vi "Write Configuration File.vi"(8 "error in (no error)":errorcluster, 11 "Inst.RP100 in":refnum<class "Inst.RP100.lvclass">) -> (0 "error out":errorcluster, 3 "Inst.RP100 out":refnum<class "Inst.RP100.lvclass">)   [LabVIEW 2019, in "Inst.RP100.lvlib" / "Inst.RP100.lvclass"]
uses:
  Inst.RP100.lvclass
  C:/Program Files (x86)/National Instruments/LabVIEW 2019/user.lib/LevyLab/Instrument Framework/Instrument/Instrument.lvclass
  Inst.RP100.lvclass/Inst.RP100.ctl
  <userlib>/LevyLab/Instrument Framework/Instrument/Instrument.lvclass/Instrument.ctl
  <userlib>/LevyLab/Configuration/Configuration.lvclass/Configuration.ctl
  <userlib>/LevyLab/Configuration/Write Section.vi
  <userlib>/LevyLab/Instrument Framework/Instrument/Instrument.lvclass
  C:/Program Files (x86)/National Instruments/LabVIEW 2019/vi.lib/JKI/JKI SMO/SMO/SMO.lvclass
  <vilib>/JKI/JKI SMO/SMO/Protected/ThisLevelClassName.vi
  <userlib>/LevyLab/Instrument Framework/Instrument Types/Strain/Instrument.Strain.lvclass
  <userlib>/LevyLab/Configuration/Configuration.lvclass
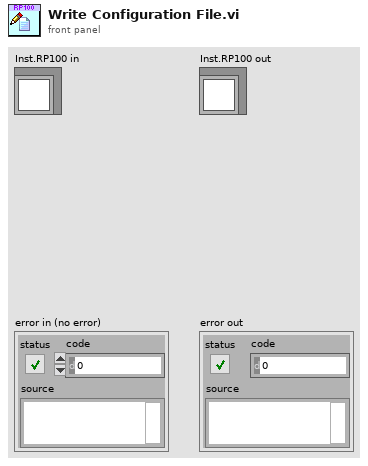
[diagram p1: front panel]
types:
  T1 = typedef "Inst.RP100.lvlib/Inst.RP100.lvclass/Inst.RP100.Configuration--Cluster.ctl" = cluster{"Example Setting 1":dbl, "Example Setting 2":dbl, "Example Setting 3":string}
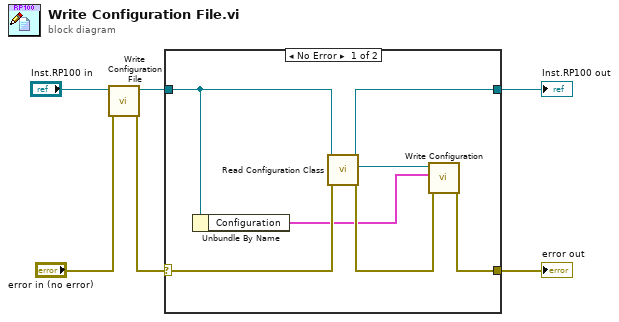
[diagram p0: block diagram]
diagram:
  n1 = call-parent "Write Configuration File.vi"("error in (no error)"="error in (no error)", "Instrument in"="Inst.RP100 in") -> ("error out"=w3:errorcluster, "Instrument out"=w1:refnum<class "Inst.RP100.lvclass">)  [unwired: 8 in]
  n2 = case shown="No Error" w3 {
    selector: w3 -> [w9 w15]
    tunnel: w1 -> [w8 w14]
    tunnel: [w12 w14] -> w6
    tunnel: [w11 w15] -> w5
    frame No Error {
      n3 = Unbundle By Name(w8) -> ("Configuration"=w7:T1)
      n4 = call <userlib>:"Read Configuration Class.vi"("error in (no error)"=w9, "Instrument in"=w8) -> ("error out"=w13:errorcluster, "Configuration"=w10:refnum<class "Configuration.lvclass">, "Instrument out"=w12:refnum<class "Inst.RP100.lvclass">)  [unwired: 7 in]
      n5 = call <userlib>:"Write Configuration.vi"("error in (no error)"=w13, "Variant"=w7, "Configuration in"=w10) -> ("error out"=w11:errorcluster)  [unwired: 7 in, 1 out]
    }
    frame Error {
    }
  }
  "Inst.RP100 out" <- w6
  "error out" <- w5
